vi "Iterate Counters.vi"(1 "Inj Event Boolean State Data":T1) -> (0 "Inj Capture Core Boolean State Data out":T1)   [LabVIEW 2015]
uses:
  Types/Injection Capture Core Boolean State Data.ctl
  <instrlib>/_niInstr/Basic Elements/v1/FPGA/Private/Count Up U8.vi
  <instrlib>/_niInstr/Basic Elements/v1/FPGA/Private/Count Up U16.vi
  <instrlib>/_niInstr/Basic Elements/v1/FPGA/Private/Count Up U32.vi
  <instrlib>/_niInstr/Basic Elements/v1/FPGA/niInstr Basic Elements v1 FPGA.lvlib
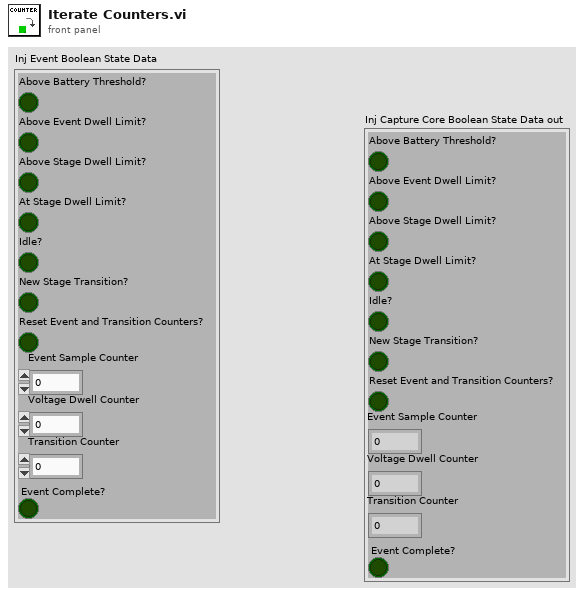
[diagram p1: front panel]
types:
  T1 = typedef "Injection Capture Core Boolean State Data.ctl" = cluster{"Above Battery Threshold?":bool, "Above Event Dwell Limit?":bool, "Above Stage Dwell Limit?":bool, "At Stage Dwell Limit?":bool, "Idle?":bool, "New Stage Transition?":bool, "Reset Event and Transition Counters?":bool, "Event Sample Counter":u16, "Voltage Dwell Counter":u32, "Transition Counter":u8, "Event Complete?":bool}
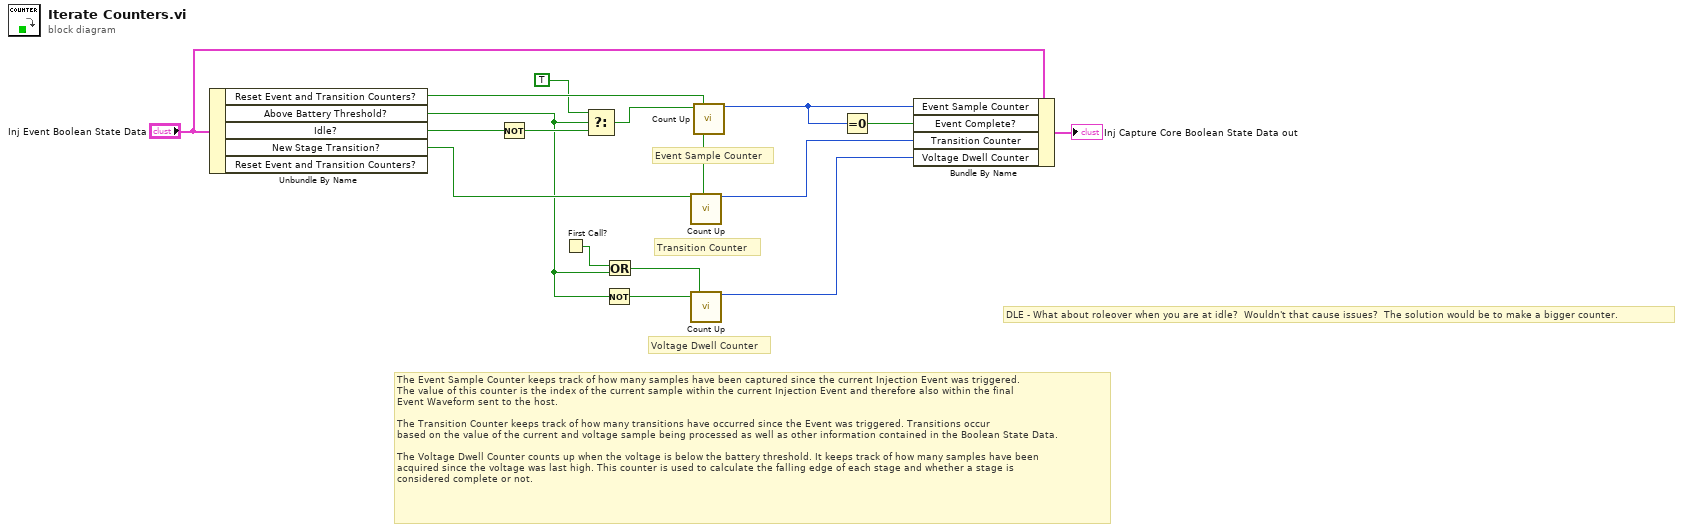
[diagram p0: block diagram]
diagram:
  # "DLE - What about roleover when you are at idle?  Wouldn't that cause issues?  The solution would be to make a bigger counter."
  # "The Event Sample Counter keeps track of how many samples have been captured since the current Injection Event was triggered.\nThe value of this counter is the index of the current sample within the current Injection Event and therefore also within the final \nEvent Waveform sent to the host.\n\nThe Transition Counter keeps track of how many transitions have occurred since the Event was triggered. Transitions occur\nbased on the value of the current and voltage sample being processed as well as other information contained in the Boolean State Data.\n\nThe Voltage Dwell Counter counts up when the voltage is below the battery threshold. It keeps track of how many samples have been \nacquired since the voltage was last high. This counter is used to calculate the falling edge of each stage and whether a stage is \nconsidered complete or not."
  # "Transition Counter"
  # "Voltage Dwell Counter"
  # "Event Sample Counter"
  n1 = Unbundle By Name("Inj Event Boolean State Data") -> ("Reset Event and Transition Counters?"=w16:bool, "Above Battery Threshold?"=w2:bool, "Idle?"=w13:bool, "New Stage Transition?"=w11:bool)  [unwired: 1 out]
  n2 = Not(x=w13) -> (.not. x?=w15:bool)
  n3 = First Call?() -> (First Call?: T/F=w1:bool)
  n4 = Select(t=TRUE, s=w2, f=w15) -> (s? t:f=w12:bool)
  n5 = Not(x=w2) -> (.not. x?=w10:bool)
  n6 = Or(x=w1, y=w2) -> (x .or. y?=w3:bool)
  n7 = call-poly <instrlib>:"Count Up.vi"("increment"=w11, "reset"=w16) -> ("count out"=w8:u8)  [unwired: 13 in]
  n8 = call-poly <instrlib>:"Count Up.vi"("increment"=w10, "reset"=w3) -> ("count out"=w7:u32)  [unwired: 13 in]
  n9 = call-poly <instrlib>:"Count Up.vi"("increment"=w12, "reset"=w16) -> ("count out"=w5:u16)  [unwired: 13 in]
  n10 = Equal To 0?(x=w5) -> (x = 0?=w4:bool)
  n11 = Bundle By Name(cluster="Inj Event Boolean State Data", "Event Sample Counter"=w5, "Event Complete?"=w4, "Transition Counter"=w8, "Voltage Dwell Counter"=w7) -> (→"Inj Capture Core Boolean State Data out":T1)
